vi "ACT L_bank_Control_05.vi"(0 "SI804.lvclass in":refnum<class "SI804.lvclass">, 1 "3 JSA20 DT102\nXA01":bool, 2 "3 JSA20 DT101\nXA01":bool, 3 "3 JSA20 DT103\nXA01":bool, 5 "error in":errorcluster) -> (14 "SI804.lvclass out":refnum<class "SI804.lvclass">, 15 "ACT-Ctrl\nL-bank insertion":bool, 16 "ACT-Control M/A":bool, 17 "ACT-Ctrl\nL-bank withdrawal":bool, 19 "error out":errorcluster)   [LabVIEW 2022 SP3, in "SI804.lvclass"]
uses:
  SI804.lvclass
  SI804.lvclass/SI804.ctl
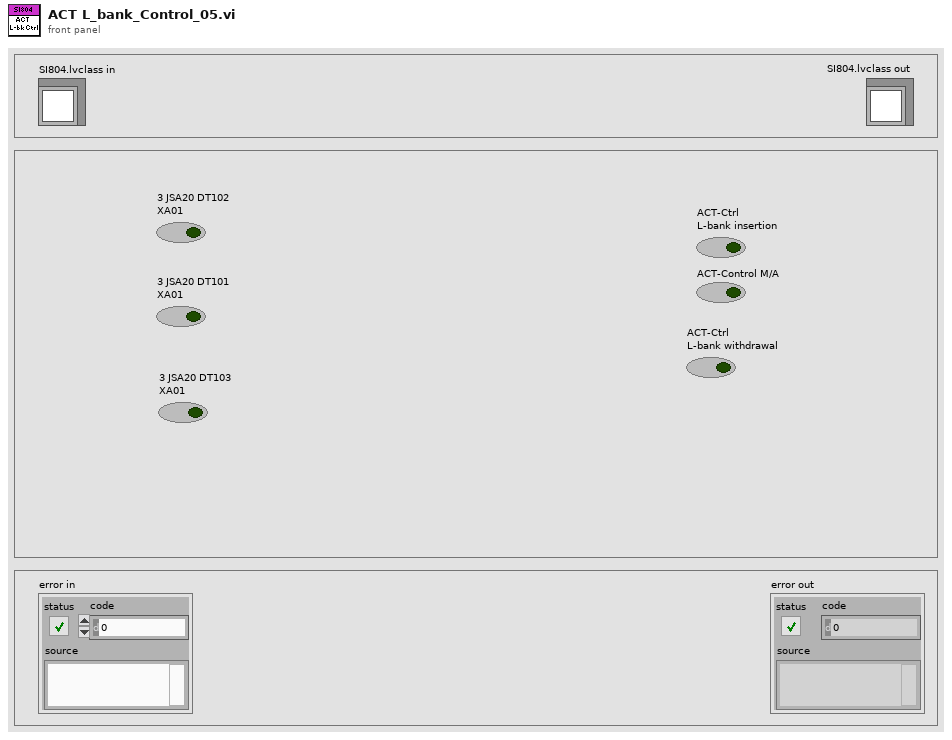
[diagram p1: front panel]
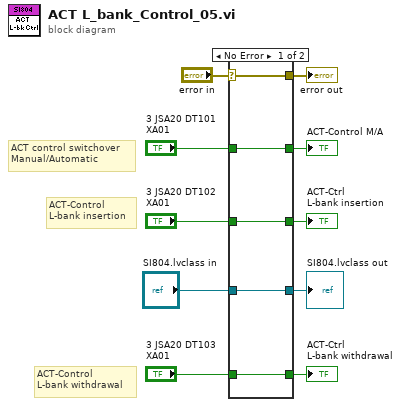
[diagram p0: block diagram]
diagram:
  # "ACT-Control\nL-bank withdrawal"
  # "ACT control switchover\nManual/Automatic"
  # "ACT-Control\nL-bank insertion"
  n1 = case shown="No Error" "error in" {
    selector: "error in" -> [w11 w16]
    tunnel: "3 JSA20 DT102\nXA01" -> [w15 _]
    tunnel: "3 JSA20 DT101\nXA01" -> [w14 _]
    tunnel: "3 JSA20 DT103\nXA01" -> [w13 _]
    tunnel: [w15 _] -> w6
    tunnel: [w14 _] -> w4
    tunnel: [w13 _] -> w5
    tunnel: "SI804.lvclass in" -> [w12 w17]
    tunnel: [w12 w17] -> w2
    tunnel: [w11 w16] -> w1
    frame No Error {
    }
    frame Error {
    }
  }
  "ACT-Ctrl\nL-bank insertion" <- w6
  "ACT-Ctrl\nL-bank withdrawal" <- w5
  "ACT-Control M/A" <- w4
  "SI804.lvclass out" <- w2
  "error out" <- w1
